vi "Monitor Transmit and Receive Messages.vi"() -> ()   [LabVIEW 2019]
doc: "This program opens the specified card, finds the first compatible core, builds a transmit schedule using transmit interval information, and creates filters for two receive messages. It also enables the Sequential Monitor to record transmitted and received messages."
uses:
  <instrlib>/BTI429Lib/Public/Controls/429 Record.ctl
  <instrlib>/BTICardLib/Private/Initialize By Card Number and Core Number.vi
  <instrlib>/BTICardLib/Private/Configure Core From XML.vi
  <instrlib>/BTI429Lib/Private/Tx/Configure/Configure Tx Channel From XML.vi
  <instrlib>/BTI429Lib/Private/Rx/Configure/Configure Rx Channel From XML.vi
  <instrlib>/BTI429Lib/Private/Core/Action-Status/Start All Channels.vi
  <instrlib>/BTI429Lib/Private/Core/Action-Status/Stop All Channels.vi
  <instrlib>/BTICardLib/BTICardLV.lvlib
  <instrlib>/BTI429Lib/BTI429LV.lvlib
panel:
  out "rx channel number":i32
  out "tx channel number":i32
  out "core number":i32
  in  "Rx Channel XML Configuration File":string="Rx Channel Config.xml"
  in  "Tx Channel XML Configuration File":string="Tx Channel Config.xml"
  out "record out":T1 {"type" format="%04x"; "timestamp" format="%08x"; "msgact" format="%04x"; "data" format="%08x"; "timestamph" format="%08x"}
  in  "Core Configuration File":string="Core Config.xml"
  in  "stop":bool
  out "error out":errorcluster
  in  "Card Number":i32
  # "ARINC 429: Monitor Transmit and Receive Messages"
  # "©2016 Astronics Ballard Technology"
  # "This program opens the specified card, finds the first compatible core, builds a transmit schedule using transmit interval information, and creates filters for two receive messages.  It also enables the Sequential Monitor to record transmitted and received messages."
  # "Always Stop the card\nand Close the card when\ndone. Otherwise, the hardware\ncontinues to operate."
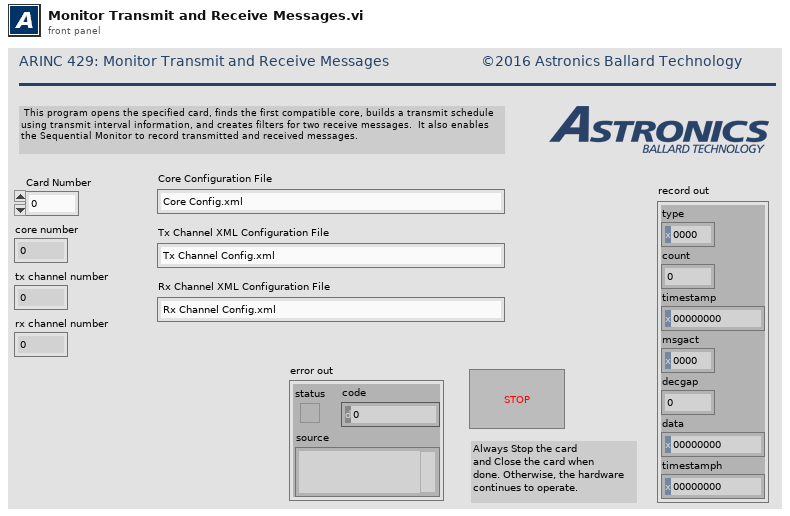
[diagram p1: front panel]
types:
  T1 = typedef "BTI429LV.lvlib/429 Record.ctl" = cluster{"type":u16, "count":u16, "timestamp":u32, "msgact":u16, "decgap":u16, "data":u32, "timestamph":u32}
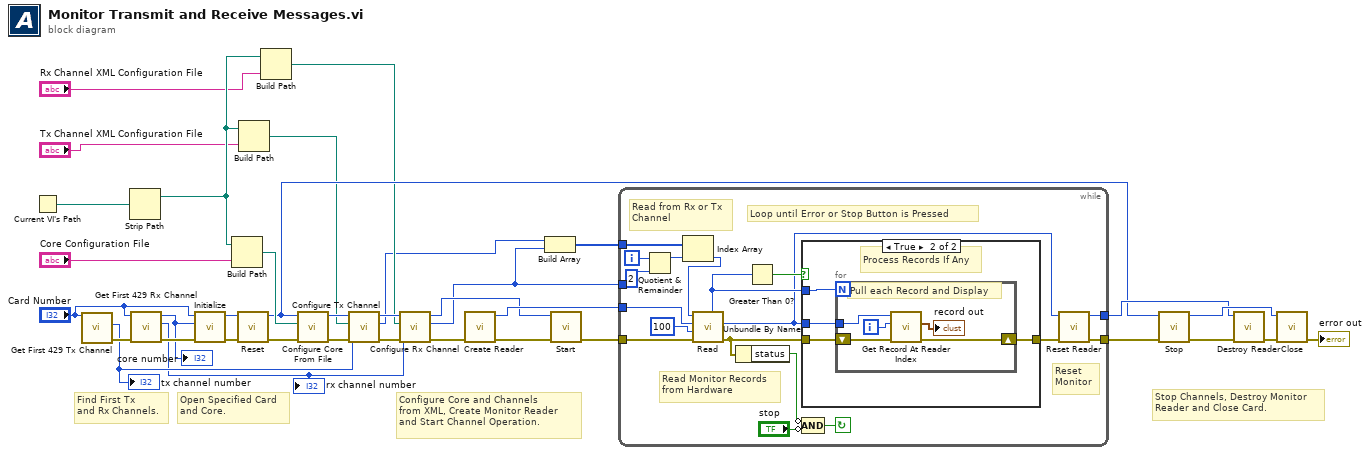
[diagram p0: block diagram]
diagram:
  # "Find First Tx \nand Rx Channels."
  # "Stop Channels, Destroy Monitor\nReader and Close Card."
  # "Configure Core and Channels \nfrom XML, Create Monitor Reader \nand Start Channel Operation."
  # "Open Specified Card\nand Core."
  n1 = Current VI's Path() -> (path=w32:path)
  n2 = call "Get First 429 Tx Channel.vi"("Card Number"="Card Number") -> ("error out"=w9:errorcluster, "Channel Number"=w6:i32)  [unwired: 8 in, 1 out]
  "tx channel number" <- w6
  n3 = Strip Path(path=w32) -> (stripped path=w20:path)  [unwired: 1 out]
  n4 = call "Get First 429 Rx Channel.vi"("error in (no error)"=w9, "Card Number"="Card Number") -> ("error out"=w8:errorcluster, "Channel Number"=w5:i32, "Core Number"=w4:i32)  [unwired: 7 in]
  "core number" <- w4
  "rx channel number" <- w5
  n5 = call-poly <instrlib>:"Initialize.vi"("error in (no error)"=w8, "core number"=w4, "card number"="Card Number") -> ("error out"=w22:errorcluster, "core handle out"=w23:u64)  [unwired: 7 in]
  n6 = Build Path(base path=w20, name or relative path="Core Configuration File") -> (appended path=w31:path)
  n7 = call <instrlib>:"Reset.vi"("error in (no error)"=w22, "core handle in"=w23) -> ("error out"=w24:errorcluster, "core handle out"=w21:u64)  [unwired: 8 in]
  n8 = Build Path(base path=w20, name or relative path="Tx Channel XML Configuration File") -> (appended path=w11:path)
  n9 = Build Path(base path=w20, name or relative path="Rx Channel XML Configuration File") -> (appended path=w10:path)
  n10 = call-poly <instrlib>:"Configure Core From File.vi"("error in (no error)"=w24, "configuration file path"=w31, "core handle in"=w21) -> ("error out"=w17:errorcluster, "core handle out"=w14:u64)  [unwired: 7 in]
  n11 = call-poly <instrlib>:"Configure Tx Channel.vi"("error in (no error)"=w17, "channel number in"=w6, "configuration file path"=w11, "core handle in"=w14) -> ("error out"=w16:errorcluster, "channel handle out"=w3:u64, "core handle out"=w13:u64)  [unwired: 5 in]
  n12 = call-poly <instrlib>:"Configure Rx Channel.vi"("error in (no error)"=w16, "channel number in"=w5, "configuration file path"=w10, "core handle in"=w13) -> ("error out"=w15:errorcluster, "channel handle out"=w2:u64, "core handle out"=w12:u64)  [unwired: 5 in]
  n13 = call <instrlib>:"Create Reader.vi"("error in (no error)"=w15) -> ("error out"=w29:errorcluster, "reader handle out"=w33:u64)  [unwired: 9 in]
  n14 = Build Array(w3, w2) -> (w1:u64[])
  n15 = call-poly <instrlib>:"Start.vi"("error in (no error)"=w29, "core handle in"=w12) -> ("error out"=w34:errorcluster)  [unwired: 8 in, 1 out]
  n16 = while {
    tunnel: [w46] -> w35
    tunnel: w33 -> [w51]
    tunnel: w34 -> [w52]
    tunnel: w2 -> [_]
    tunnel: [w42] -> w25
    tunnel: w1 -> [w38]
    i -> [w41]
    stop <- w53 continue-if-true
    # "Read from Rx or Tx\nChannel"
    # "Reset\nMonitor"
    # "Read Monitor Records\nfrom Hardware"
    # "Loop until Error or Stop Button is Pressed"
    n17 = Quotient & Remainder(x=w41, y=2) -> (x-y*floor(x/y)=w39:i32)  [unwired: 1 out]
    n18 = Index Array(array=w38, index=w39) -> (element=w37:u64)
    n19 = call <instrlib>:"Read.vi"("error in (no error)"=w52, "max records to read"=100, "reader handle in"=w51, "channel handle in"=w37) -> ("error out"=w44:errorcluster, "reader handle out"=w45:u64, "records read"=w47:i32)  [unwired: 3 in, 2 out]
    n20 = Unbundle By Name(w44) -> ("status"=w54:bool)
    n21 = Greater Than 0?(x=w47) -> (x > 0?=w48:bool)
    n22 = case shown="True" w48 {
      tunnel: w45 -> [_ w59]
      tunnel: w47 -> [_ w58]
      tunnel: w44 -> [w55 w56]
      tunnel: [w55 w57] -> w43
      frame False {
      }
      frame True {
        # "Process Records If Any"
        n23 = for {
          N: w58 -> [_]
          tunnel: w59 -> [w64]
          shift-right: [w62] -> w57
          shift-left: w56 -> [w61]
          i -> [w63]
          # "Pull each Record and Display"
          n24 = call <instrlib>:"Get Record At Reader Index.vi"("error in (no error)"=w61, "record index"=w63, "reader handle in"=w64) -> ("error out"=w62:errorcluster, "record out"=→"record out":T1)  [unwired: 6 in, 1 out]
        }
      }
    }
    n25 = Compound Arithmetic op=AND(invert w54, invert "stop") -> (w53:bool)
    n26 = call <instrlib>:"Reset Reader.vi"("error in (no error)"=w43, "reader handle in"=w45) -> ("error out"=w46:errorcluster, "reader handle out"=w42:u64)  [unwired: 8 in]
  }
  n27 = call-poly <instrlib>:"Stop.vi"("error in (no error)"=w35, "core handle in"=w21) -> ("error out"=w28:errorcluster, "core handle out"=w26:u64)  [unwired: 8 in]
  n28 = call <instrlib>:"Destroy Reader.vi"("error in (no error)"=w28, "reader handle in"=w25) -> ("error out"=w27:errorcluster)  [unwired: 8 in, 1 out]
  n29 = call <instrlib>:"Close.vi"("error in (no error)"=w27, "core handle in"=w26) -> ("error out"=→"error out":errorcluster)  [unwired: 8 in, 1 out]
